vi "Safety_Check.vi"(1 "Adam Loop Count":i32, 2 "Ch Names":string[](array[string]), 3 "Values":dbl[](array[numeric]) format="%.2f") -> ()   [LabVIEW 2010]
uses:
  ADAM Client/Sub VIs/ADAM Controls/Update_scan_value.ctl
  Anemometry/Anemometry Sub Vis/Globals/Gas_management_global.vi
  ADAM_Global.vi
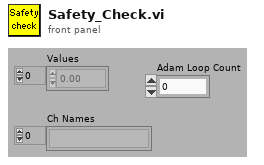
[diagram p1: front panel]
types:
  T1 = enum16{"On", "Off", "Always On", "Always Off", "Delete"}
  T2 = cluster{"Channel name":string, "Set value of A to":dbl, "Set value of B to":dbl, "Set value of C to":dbl, "Set value of D to":dbl}
  T3 = typedef "Update_scan_value.ctl" = cluster{"Channel Name":string, "New Value":dbl}
  T4 = enum16{"Append to Global", "Read Global then Clear"}
  T5 = typedef "LVDateTimeRec.ctl" = cluster{"fractional second":dbl, "second":i32, "minute":i32, "hour":i32, "day of month":i32, "month":i32, "year":i32, "day of week":i32, "day of year":i32, "DST":i32}
  T6 = cluster{"Channel name":string, "Set value of A to":dbl, "Set value of B to":dbl, "Set value of C to":dbl, "Set value of D to":dbl}[]
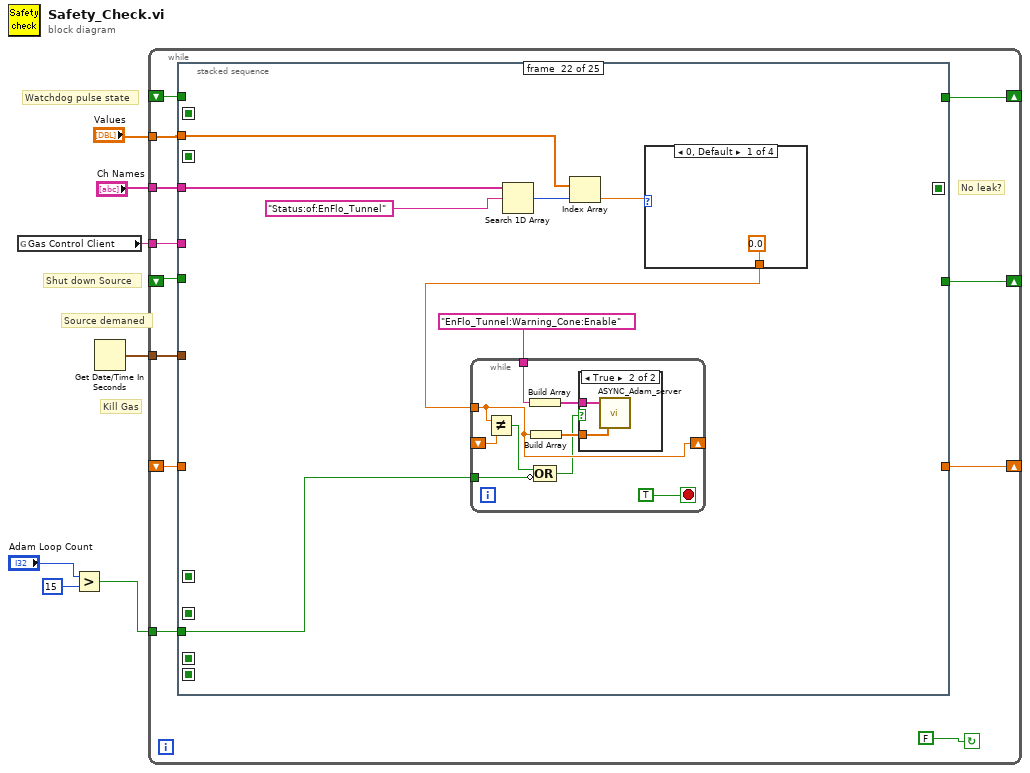
[diagram p0: block diagram]
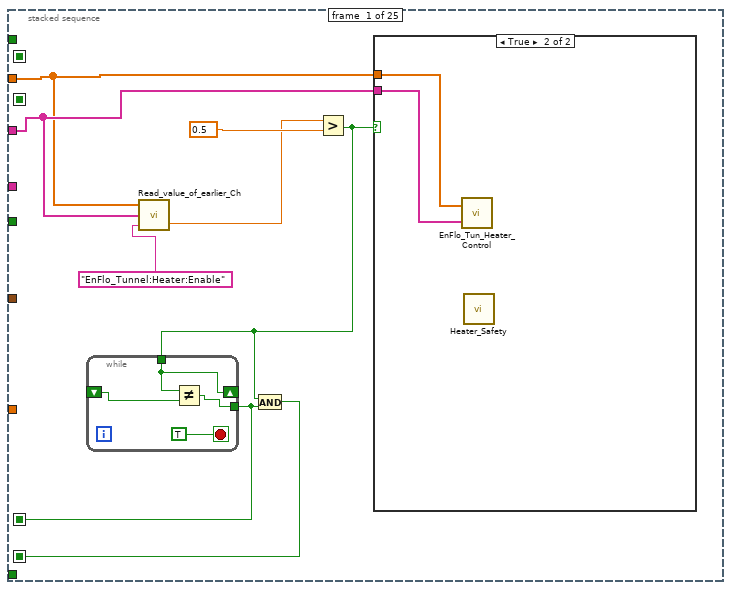
[diagram p2: hidden frame]
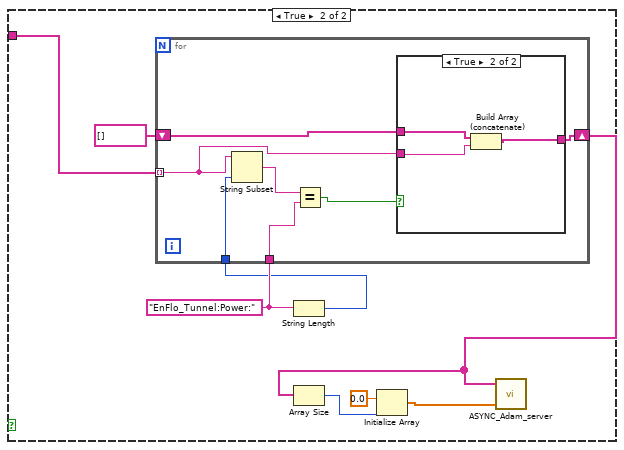
[diagram p5: hidden frame]
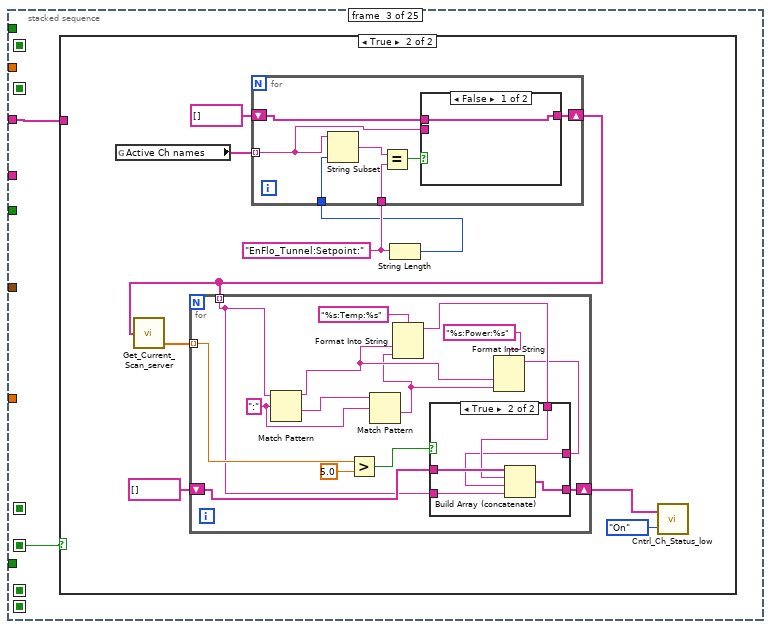
[diagram p7: hidden frame]
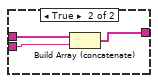
[diagram p10: hidden frame]
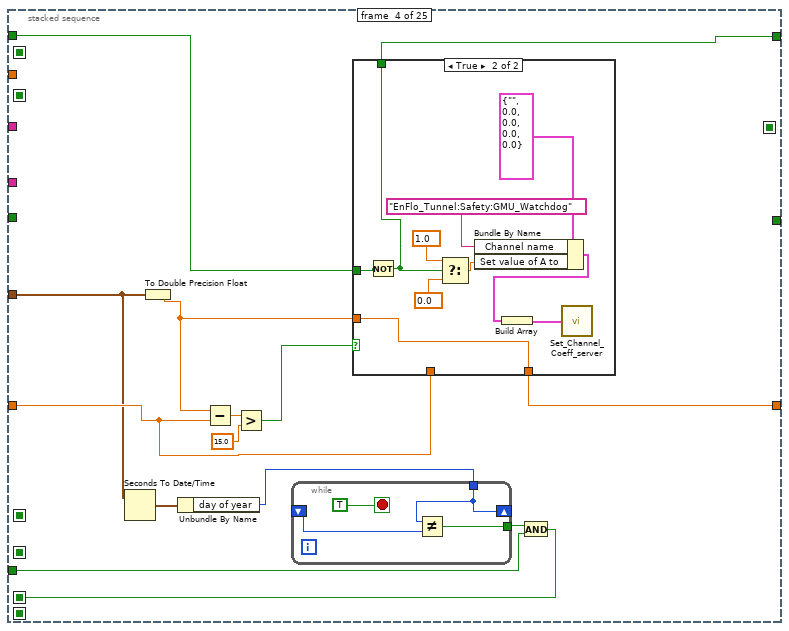
[diagram p11: hidden frame]
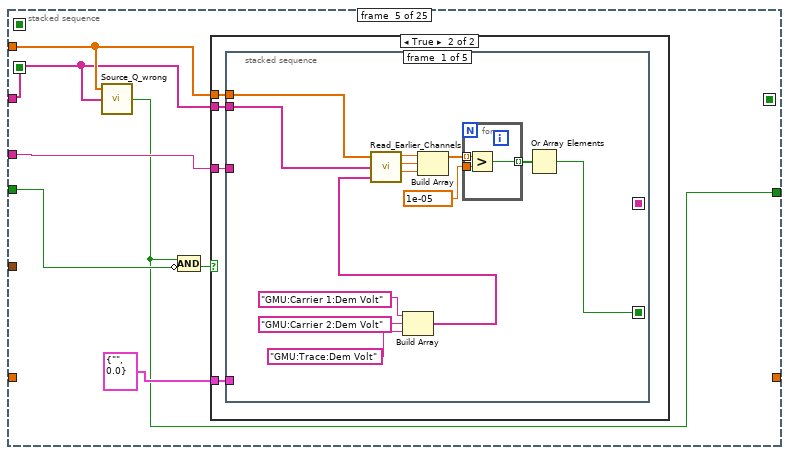
[diagram p13: hidden frame]
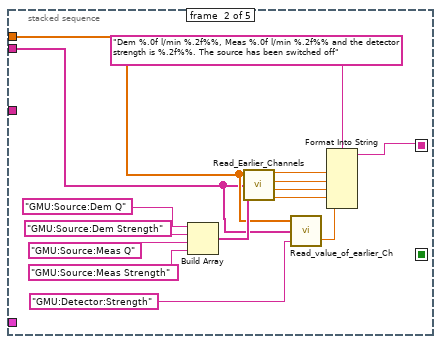
[diagram p15: hidden frame]
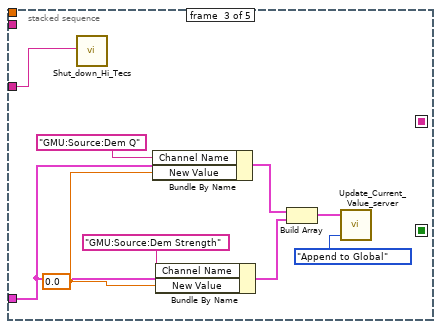
[diagram p16: hidden frame]
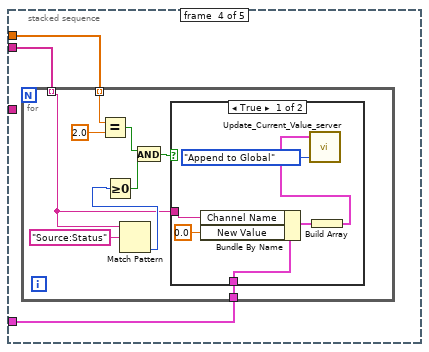
[diagram p17: hidden frame]
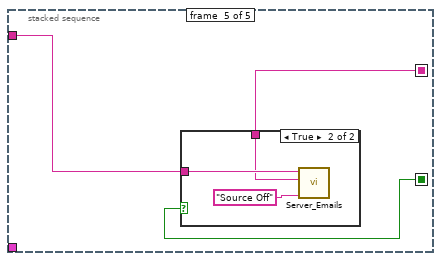
[diagram p19: hidden frame]
diagram:
  # "Shut down Source"
  # "Source demaned"
  # "Watchdog pulse state"
  # "Kill Gas"
  n1 = global read "Gas_management_global.vi" "Gas Control Client"() -> (w5:string)
  n2 = Greater?(x="Adam Loop Count", y=15) -> (0:w2:bool)
  n3 = Get Date/Time In Seconds() -> (seconds since 1Jan1904=w1:timestamp)
  n4 = while {
    shift-left: _ -> [w14]
    shift-right: [w13] -> _
    shift-left: _ -> [w16]
    shift-right: [w15] -> _
    tunnel: w5 -> [w18]
    tunnel: "Ch Names" -> [w19]
    tunnel: "Values" -> [w17]
    shift-right: [w11] -> _
    shift-left: _ -> [w10]
    tunnel: w2 -> [w9]
    tunnel: w1 -> [w8]
    stop <- FALSE continue-if-true
    # "No leak?"
    n5 = stacked-sequence {
      seq-local: [_ _ _ _ _ _ _ w234 _ _ _ _ _ _ _ _ _ _ _ _ _ _ _ _ _] -> [_ _ _ _ _ _ _ _ _ _ _ _ _ _ _ _ _ w505 _ _ _ _ _ _ _]
      seq-local: [w21 _ _ _ _ _ _ _ _ _ _ _ _ _ _ _ _ _ _ _ _ _ _ _ _] -> [_ _ w56 _ _ _ _ _ _ _ _ _ _ _ _ _ _ _ _ _ _ _ _ _ _]
      seq-local: [w20 _ _ _ _ _ _ _ _ _ _ _ _ _ _ _ _ _ _ _ _ _ _ _ _] -> [_ w34 _ _ _ _ _ _ _ _ _ _ _ _ _ _ _ _ _ _ _ _ _ _ _]
      seq-local: [_ _ _ w98 _ _ _ _ _ _ _ _ _ _ _ _ _ _ _ _ _ _ _ _ _] -> [_ _ _ _ _ _ _ _ _ _ _ _ _ _ _ w441 _ _ _ _ _ _ _ _ _]
      seq-local: [_ _ _ _ _ _ _ _ _ _ _ _ _ _ _ _ _ _ _ w534 _ _ _ _ _] -> [_ _ _ _ _ _ _ _ _ _ _ _ _ _ _ _ _ _ _ _ w560 _ _ _ _]
      seq-local: [_ _ _ _ _ _ _ _ _ _ _ _ _ _ _ _ _ _ _ _ w552 _ _ _ _] -> [_ _ _ _ _ _ _ _ _ _ _ _ _ _ _ _ _ _ _ _ _ _ _ w665 _]
      seq-local: [_ _ _ _ _ _ _ _ _ w276 _ _ _ _ _ _ _ _ _ _ _ _ _ _ _] -> [_ _ _ _ _ _ _ _ _ _ w303 _ _ _ _ _ _ _ _ _ _ _ _ _ _]
      tunnel: w19 -> [w25 w35 w55 _ w128 w207 w218 w235 w249 w277 _ w352 w380 w404 w423 w451 w476 w503 w521 w535 w561 w616 w635 _ w685]
      tunnel: w18 -> [_ _ _ _ w133 _ w217 _ _ _ _ _ _ _ _ _ _ _ _ _ _ _ _ _ _]
      tunnel: w17 -> [w24 _ _ _ w129 w203 w219 w236 w250 w278 _ w353 w381 w405 w424 w452 w477 w504 w522 w536 w562 w617 w636 _ w684]
      tunnel: w16 -> [_ _ _ w110 _ _ _ _ _ _ _ _ _ _ _ _ _ _ _ _ _ _ _ _ _]
      tunnel: [_ _ _ w109 _ _ _ _ _ _ _ _ _ _ _ _ _ _ _ _ _ _ _ _ _] -> w15
      tunnel: w14 -> [_ _ _ _ w132 _ _ _ _ _ _ _ _ _ _ _ _ _ _ _ _ _ _ _ _]
      tunnel: [_ _ _ _ w127 _ _ _ _ _ _ _ _ _ _ _ _ _ _ _ _ _ _ _ _] -> w13
      tunnel: [_ _ _ w108 _ _ _ _ _ _ _ _ _ _ _ _ _ _ _ _ _ _ _ _ _] -> w11
      tunnel: w10 -> [_ _ _ w104 _ _ _ _ _ _ _ _ _ _ _ _ _ _ _ _ _ _ _ _ _]
      tunnel: w9 -> [_ _ _ w99 _ _ _ _ _ _ w301 _ _ _ w422 _ _ _ _ _ w553 w612 _ w664 w679]
      tunnel: w8 -> [_ _ _ w97 _ _ _ _ _ _ w304 _ w376 _ _ _ _ _ _ _ _ _ _ _ _]
      frame #0 {
        n6 = call "Read_value_of_earlier_Ch.vi"("Desired Ch to Read"="EnFlo_Tunnel:Heater:Enable", "Ch names"=w25, "Present scan array"=w24) -> ("Value"=w23:dbl)  [unwired: 1 in, 1 out]
        n7 = Greater?(x=w23, y=0.5) -> (0:w22:bool)
        n8 = while {
          shift-right: [w31] -> _
          shift-left: _ -> [w30]
          tunnel: w22 -> [w31]
          tunnel: [w28] -> w20
          stop <- TRUE stop-if-true
          n9 = Not Equal?(x=w31, y=w30) -> (x != y?=w28:bool)
        }
        n10 = And(x=w22, y=w20) -> (x .and. y?=w21:bool)
        n11 = case shown="True" w22 {
          tunnel: w24 -> [_ w33]
          tunnel: w25 -> [_ w32]
          frame False {
          }
          frame True {
            n12 = call "EnFlo_Tun_Heater_Control.vi"("Ch Names"=w32, "Values"=w33) -> ()  [unwired: 1 out]
            n13 = call "Heater_Safety.vi"() -> ()  [unwired: 3 in, 5 out]
          }
        }
      }
      frame #1 {
        n14 = case shown="False" w34 {
          tunnel: w35 -> [_ w43]
          frame False {
          }
          frame True {
            w42 = "EnFlo_Tunnel:Power:"
            n15 = String Length(string=w42) -> (length=w41:i32)
            n16 = for {
              shift-right: [w45] -> w37
              shift-left: string[] [] -> [w46]
              tunnel: w43 -> [w49] mode=indexing
              tunnel: w41 -> [w50]
              tunnel: w42 -> [w47]
              n17 = String Subset(string=w49, length (rest)=w50) -> (substring=w48:string)  [unwired: 1 out]
              n18 = Equal?(x=w48, y=w47) -> (x = y?=w44:bool)
              n19 = case shown="True" w44 {
                tunnel: w49 -> [_ w54]
                tunnel: w46 -> [w51 w52]
                tunnel: [w51 w53] -> w45
                frame False {
                }
                frame True {
                  n20 = Build Array (concatenate)(w52, w54) -> (w53:string[])
                }
              }
            }
            n21 = Array Size(array=w37) -> (size(s)=w38:i32)
            n22 = Initialize Array(0.0 ("element"), w38) -> (w36:dbl[])
            n23 = call "ASYNC_Adam_server.vi"("Values"=w36, "Channel Names"=w37) -> ()  [unwired: 1 in, 3 out]
          }
        }
      }
      frame #2 {
        n24 = case shown="True" w56 {
          tunnel: w55 -> [_ _]
          frame False {
          }
          frame True {
            w64 = "EnFlo_Tunnel:Setpoint:"
            n25 = global read "ADAM_Global.vi" "Active Ch names"() -> (w62:string[])
            n26 = String Length(string=w64) -> (length=w63:i32)
            n27 = for {
              shift-right: [w86] -> w61
              shift-left: string[] [] -> [w88]
              tunnel: w62 -> [w87] mode=indexing
              tunnel: w63 -> [w92]
              tunnel: w64 -> [w91]
              n28 = String Subset(string=w87, length (rest)=w92) -> (substring=w90:string)  [unwired: 1 out]
              n29 = Equal?(x=w90, y=w91) -> (x = y?=w89:bool)
              n30 = case shown="False" w89 {
                tunnel: w88 -> [w93 w96]
                tunnel: w87 -> [_ w95]
                tunnel: [w93 w94] -> w86
                frame False {
                }
                frame True {
                  n31 = Build Array (concatenate)(w96, w95) -> (w94:string[])
                }
              }
            }
            n32 = call "Get_Current_Scan_server.vi"("Desired Channels"=w61) -> ("Numerical Values"=w60:dbl[])  [unwired: 2 out]
            n33 = for {
              tunnel: w61 -> [w66] mode=indexing
              tunnel: w60 -> [w73] mode=indexing
              shift-right: [w67] -> w58
              shift-left: string[] [] -> [w71]
              w78 = ":" ("regular expression")
              n34 = Match Pattern(string=w66, regular expression=w78) -> (before substring=w75:string, after substring=w79:string)  [unwired: 3 out]
              n35 = Greater?(x=w73, y=5.0) -> (0:w70:bool)
              n36 = Match Pattern(string=w79, regular expression=w78) -> (after substring=w74:string)  [unwired: 4 out]
              n37 = Format Into String(format string="%s:Temp:%s", w75, w74) -> (resulting string=w69:string)  [unwired: 2 in, 1 out]
              n38 = Format Into String(format string="%s:Power:%s", w75, w74) -> (resulting string=w68:string)  [unwired: 2 in, 1 out]
              n39 = case shown="True" w70 {
                tunnel: w71 -> [w80 w85]
                tunnel: w69 -> [_ w84]
                tunnel: w68 -> [_ w83]
                tunnel: [w80 w82] -> w67
                tunnel: w66 -> [_ w81]
                frame False {
                }
                frame True {
                  n40 = Build Array (concatenate)(w85, w84, w83, w81) -> (w82:string[])
                }
              }
            }
            n41 = call "Cntrl_Ch_Status_low.vi"("Mode"=T1."On", "Channel names"=w58) -> ()  [unwired: 1 out]
          }
        }
      }
      frame #3 {
        n42 = Seconds To Date/Time(time stamp (now)=w97) -> (date time rec=w102:T5)  [unwired: 1 in]
        n43 = To Double Precision Float(number=w97) -> (double precision float=w107:dbl)
        n44 = Unbundle By Name(w102) -> ("day of year"=w101:i32)
        n45 = Subtract(x=w107, y=w104) -> (x-y=w106:dbl)
        n46 = Greater?(x=w106, y=15.0) -> (0:w103:bool)
        n47 = while {
          shift-right: [w114] -> _
          shift-left: _ -> [w113]
          tunnel: w101 -> [w114]
          tunnel: [w112] -> w100
          stop <- TRUE stop-if-true
          n48 = Not Equal?(x=w114, y=w113) -> (x != y?=w112:bool)
        }
        n49 = case shown="True" w103 {
          tunnel: w110 -> [w115 w119]
          tunnel: [w115 w118] -> w109
          tunnel: [w116 w117] -> w108
          tunnel: w107 -> [_ w117]
          tunnel: w104 -> [w116 _]
          frame False {
          }
          frame True {
            n50 = Not(x=w119) -> (.not. x?=w118:bool)
            n51 = Select(t=1.0 ("Suction"), s=w118, f=0.0 ("Suction")) -> (s? t:f=w122:dbl)
            n52 = Bundle By Name(cluster=T2 {"Channel name"="", "Set value of A to"=0.0, "Set value of B to"=0.0, "Set value of C to"=0.0, "Set value of D to"=0.0}, "Channel name"="EnFlo_Tunnel:Safety:GMU_Watchdog" ("Desired Ch to Read"), "Set value of A to"=w122) -> (w126:T2)
            n53 = Build Array(w126) -> (w121:T6)
            n54 = call "Set_Channel_Coeff_server.vi"("Set Array"=w121) -> ()
          }
        }
        n55 = And(x=w100, y=w99) -> (x .and. y?=w98:bool)
      }
      frame #4 {
        n56 = call "Source_Q_wrong.vi"("Ch Names"=w128, "Values"=w129) -> ("Gas Error?"=w127:bool)  [unwired: 1 out]
        n57 = Compound Arithmetic op=AND(w127, invert w132) -> (w131:bool)
        n58 = case shown="True" w131 {
          tunnel: w133 -> [_ w137]
          tunnel: w129 -> [_ w136]
          tunnel: w128 -> [_ w135]
          tunnel: T3 {"Channel Name"="", "New Value"=0.0} ("Update Scan Value Cluster") -> [_ w134]
          frame False {
          }
          frame True {
            n59 = stacked-sequence {
              seq-local: [_ w167 _ _ _] -> [_ _ _ _ w197]
              seq-local: [w138 _ _ _ _] -> [_ _ _ _ w196]
              tunnel: w137 -> [_ _ w170 _ w198]
              tunnel: w136 -> [w148 w157 _ w179 _]
              tunnel: w135 -> [w149 w156 _ w180 _]
              tunnel: w134 -> [_ _ w169 w178 _]
              frame #0 {
                n60 = Build Array("GMU:Carrier 1:Dem Volt", "GMU:Carrier 2:Dem Volt", "GMU:Trace:Dem Volt") -> (w150:string[])
                n61 = call "Read_Earlier_Channels.vi"("Present scan array"=w148, "Ch names"=w149, "Desired Channels"=w150) -> ("Index 0"=w144:dbl, "Index 1"=w143:dbl, "Index 2"=w142:dbl)  [unwired: 3 out]
                n62 = Build Array(w144, w143, w142) -> (w141:dbl[])
                n63 = for {
                  tunnel: w141 -> [w153] mode=indexing
                  tunnel: 1e-05 -> [w152]
                  tunnel: [w151] -> w139 mode=indexing
                  n64 = Greater?(x=w153, y=w152) -> (0:w151:bool)
                }
                n65 = Or Array Elements(Boolean array=w139) -> (logical OR=w138:bool)
              }
              frame #1 {
                n66 = Build Array("GMU:Source:Dem Q", "GMU:Source:Dem Strength", "GMU:Source:Meas Q", "GMU:Source:Meas Strength") -> (w162:string[])
                n67 = call "Read_Earlier_Channels.vi"("Present scan array"=w157, "Ch names"=w156, "Desired Channels"=w162) -> ("Index 0"=w161:dbl, "Index 1"=w160:dbl, "Index 2"=w159:dbl, "Index 3"=w158:dbl)  [unwired: 2 out]
                n68 = call "Read_value_of_earlier_Ch.vi"("Desired Ch to Read"="GMU:Detector:Strength", "Ch names"=w156, "Present scan array"=w157) -> ("Value"=w154:dbl)  [unwired: 1 in, 1 out]
                n69 = Format Into String(format string="Dem %.0f l/min %.2f%%, Meas %.0f l/min %.2f%% and the detector strength is %.2f%%. The source has been switched off" ("Format String"), w161, w160, w159, w158, w154) -> (resulting string=w167:string)  [unwired: 2 in, 1 out]
              }
              frame #2 {
                w171 = 0.0 ("Bundle Element")
                n70 = call "Shut_down_Hi_Tecs.vi"("Client Name"=w170) -> ()  [unwired: 6 out]
                n71 = Bundle By Name(cluster=w169, "Channel Name"="GMU:Source:Dem Q", "New Value"=w171) -> (w176:T3)
                n72 = Bundle By Name(cluster=w169, "Channel Name"="GMU:Source:Dem Strength", "New Value"=w171) -> (w177:T3)
                n73 = Build Array(w176, w177) -> (w173:T3[])
                n74 = call "Update_Current_Value_server.vi"("Mode"=T4."Append to Global", "Update array in"=w173) -> ()  [unwired: 1 in, 1 out]
              }
              frame #3 {
                n75 = for {
                  tunnel: w180 -> [w181] mode=indexing
                  tunnel: w179 -> [w187] mode=indexing
                  tunnel: w178 -> [w182]
                  n76 = Equal?(x=w187, y=2.0) -> (x = y?=w184:bool)
                  n77 = Match Pattern(string=w181, regular expression="Source:Status") -> (offset past match=w188:i32)  [unwired: 4 out]
                  n78 = Greater Or Equal To 0?(x=w188) -> (x >= 0?=w185:bool)
                  n79 = And(x=w184, y=w185) -> (x .and. y?=w183:bool)
                  n80 = case shown="True" w183 {
                    tunnel: w182 -> [w195 _]
                    tunnel: w181 -> [w194 _]
                    frame True {
                      n81 = Bundle By Name(cluster=w195, "Channel Name"=w194, "New Value"=0.0) -> (w192:T3)
                      n82 = Build Array(w192) -> (w191:T3[])
                      n83 = call "Update_Current_Value_server.vi"("Mode"=T4."Append to Global", "Update array in"=w191) -> ()  [unwired: 1 in, 1 out]
                    }
                    frame False {
                    }
                  }
                }
              }
              frame #4 {
                n84 = case shown="True" w196 {
                  tunnel: w198 -> [_ w201]
                  tunnel: w197 -> [_ w200]
                  frame False {
                  }
                  frame True {
                    n85 = call "Server_Emails.vi"("Client Name Contains"=w201, "Message"=w200, "Subject"="Source Off") -> ()  [unwired: 2 in, 3 out]
                  }
                }
              }
            }
          }
        }
      }
      frame #5 {
        n86 = global read "ADAM_Global.vi" "Program Hung Clients"() -> (w208:string[])
        n87 = for {
          tunnel: w208 -> [w214] mode=indexing
          tunnel: w203 -> [w216]
          tunnel: w207 -> [w215]
          tunnel: [w212] -> w206 mode=indexing
          tunnel: [w209] -> w205 mode=indexing
          n88 = call "Split_Ch_name.vi"("Ch name"=w214) -> ("Low level"=w211:string)  [unwired: 2 out]
          n89 = call "Shut_Down_Client_Demands.vi"("Ch Names"=w215, "Values"=w216, "Client Name"=w214) -> ()  [unwired: 1 out]
          n90 = Concatenate Strings(w211, ":Source:Status") -> (w212:string)
          n91 = Concatenate Strings(w211, ":Program:Sync") -> (w209:string)
        }
        n92 = Build Array (concatenate)(w206, w205) -> (w204:string[])
        n93 = call "Cntrl_Ch_Status_low.vi"("Mode"=T1."Delete", "Channel names"=w204) -> ()  [unwired: 1 out]
      }
      frame #6 {
        n94 = while {
          tunnel: w219 -> [w230]
          tunnel: w218 -> [w229]
          shift-right: [w224] -> _
          shift-left: _ -> [w225]
          tunnel: w217 -> [w222]
          stop <- FALSE continue-if-true
          n95 = call "Read_value_of_earlier_Ch.vi"("Desired Ch to Read"="GMU:Detector:Happy", "Ch names"=w229, "Present scan array"=w230) -> ("Value"=w227:dbl)  [unwired: 1 in, 1 out]
          n96 = Greater?(x=w227, y=0.5) -> (0:w224:bool)
          n97 = Compound Arithmetic op=AND(invert w224, w225) -> (w223:bool)
          n98 = case shown="True" w223 {
            tunnel: w222 -> [_ w232]
            frame False {
            }
            frame True {
              n99 = call "Server_Emails.vi"("Client Name Contains"=w232, "Message"="The GMU Gas detector IR2100 is unhappy. Please check concentrations etc. This will have turned off the gases from the outside bottle store.  You will need to repress the blue gas button after clearing the fault by purging the source with carrier gas only.", "Subject"="GMU Gas Detector Unhappy") -> ()  [unwired: 2 in, 3 out]
            }
          }
        }
        n100 = global write "ADAM_Global.vi" "Program Hung Clients"(string[] [] ("Program Hung Clients")) -> ()
      }
      frame #7 {
        n101 = while {
          tunnel: w236 -> [w245]
          tunnel: w235 -> [w244]
          shift-right: [w239] -> w234
          shift-left: _ -> [w240]
          stop <- FALSE continue-if-true
          n102 = call "Read_value_of_earlier_Ch.vi"("Desired Ch to Read"="EnFlo Lab:Leak_Detector:Happy", "Ch names"=w244, "Present scan array"=w245) -> ("Value"=w242:dbl)  [unwired: 1 in, 1 out]
          n103 = Greater?(x=w242, y=0.5) -> (0:w239:bool)
          n104 = Compound Arithmetic op=AND(invert w239, w240) -> (w238:bool)
          n105 = case shown="True" w238 {
            frame False {
            }
            frame True {
              n106 = call "Server_Emails.vi"("Client Name Contains"="EnFlo_Tunnel", "Message"="The leak detector is indicating a leak under the Enflo Tunnel. The chiller pumps should automaticaly be turned off and the cooling circuit isolated from the  University Chilled water system. The heaters should also have been disabled.", "Subject"="Leak Detected under EnFlo Tunnel") -> ()  [unwired: 2 in, 3 out]
            }
          }
        }
      }
      frame #8 {
        n107 = while {
          tunnel: w250 -> [w262]
          tunnel: w249 -> [w261]
          shift-right: [w255] -> _
          shift-left: _ -> [w251]
          stop <- FALSE continue-if-true
          w253 = 60.0 ("y")
          n108 = Decrement(x=w253) -> (x-1=w254:dbl)
          n109 = Select(t=w254, s=w251, f=w253) -> (s? t:f=w252:dbl)
          n110 = call "Read_value_of_earlier_Ch.vi"("Desired Ch to Read"="EnFlo_Tunnel:Chilled Water:Motor1 Temp", "Ch names"=w261, "Present scan array"=w262) -> ("Value"=w269:dbl)  [unwired: 1 in, 1 out]
          n111 = call "Read_value_of_earlier_Ch.vi"("Desired Ch to Read"="EnFlo_Tunnel:Chilled Water:Motor2 Temp", "Ch names"=w261, "Present scan array"=w262) -> ("Value"=w266:dbl)  [unwired: 1 in, 1 out]
          n112 = Greater?(x=w269, y=w252) -> (0:w263:bool)
          n113 = Greater?(x=w266, y=w252) -> (0:w264:bool)
          n114 = Or(x=w263, y=w264) -> (x .or. y?=w257:bool)
          n115 = call "Read_value_of_earlier_Ch.vi"("Desired Ch to Read"="EnFlo_Tunnel:Chiller_Pump:Enable", "Ch names"=w261, "Present scan array"=w262) -> ("Value"=w259:dbl)  [unwired: 1 in, 1 out]
          n116 = Greater?(x=w259, y=0.5) -> (0:w256:bool)
          n117 = And(x=w256, y=w257) -> (x .and. y?=w255:bool)
          n118 = Compound Arithmetic op=AND(w255, invert w251) -> (w268:bool)
          n119 = case shown="True" w268 {
            tunnel: w253 -> [_ w272]
            frame False {
            }
            frame True {
              n120 = Format Into String(format string="The Chilled Water Motor Temp is greater than %.0f deg C." ("Message"), w272) -> (resulting string=w271:string)  [unwired: 2 in, 1 out]
              n121 = call "Server_Emails.vi"("Client Name Contains"="EnFlo_Tunnel", "Message"=w271, "Subject"="Chilled Water Motor Temp") -> ()  [unwired: 2 in, 3 out]
            }
          }
        }
      }
      frame #9 {
        n122 = while {
          tunnel: w278 -> [w291]
          tunnel: w277 -> [w290]
          shift-right: [w286] -> _
          shift-left: _ -> [w283]
          tunnel: [w279] -> w276
          stop <- FALSE continue-if-true
          w281 = 60.0 ("y")
          w284 = "Laser:Cooling_Pump:Motor_Temp" ("Desired Ch to Read")
          n123 = Decrement(x=w281) -> (x-1=w280:dbl)
          n124 = Select(t=w280, s=w283, f=w281) -> (s? t:f=w282:dbl)
          n125 = call "Read_value_of_earlier_Ch.vi"("Desired Ch to Read"=w284, "Ch names"=w290, "Present scan array"=w291) -> ("Value"=w294:dbl)  [unwired: 1 in, 1 out]
          n126 = Greater?(x=w294, y=w282) -> (0:w285:bool)
          n127 = call "Read_value_of_earlier_Ch.vi"("Desired Ch to Read"="Laser:Cooling_Pump:Enable", "Ch names"=w290, "Present scan array"=w291) -> ("Value"=w288:dbl)  [unwired: 1 in, 1 out]
          n128 = Greater?(x=w288, y=0.5) -> (0:w279:bool)
          n129 = And(x=w279, y=w285) -> (x .and. y?=w286:bool)
          n130 = Compound Arithmetic op=AND(w286, invert w283) -> (w293:bool)
          n131 = case shown="True" w293 {
            tunnel: w281 -> [_ w297]
            tunnel: w284 -> [_ w295]
            frame False {
            }
            frame True {
              n132 = Format Into String(format string="The %s is greater than %.0f deg C." ("Message"), w295, w297) -> (resulting string=w296:string)  [unwired: 2 in, 1 out]
              n133 = call "Server_Emails.vi"("Client Name Contains"="EnFlo_Tunnel", "Message"=w296, "Subject"=w295) -> ()  [unwired: 2 in, 3 out]
            }
          }
        }
      }
      frame #10 {
        n134 = case shown="True" w303 {
          tunnel: w304 -> [_ w338]
          tunnel: [0.0 ("y") w323] -> w300
          frame False {
          }
          frame True {
            w336 = 7200.0  # Seconds
            w334 = FALSE  # All Active Channels
            n135 = To Double Precision Float(number=w338) -> (double precision float=w332:dbl)
            n136 = call "Channel_Names_and_indicies.vi"("All Active Channels"=w334, "Desired Ch Names"=string[] ["LDA Laser:Tank:Supply Temp", "LDA Laser:Tank:Return Temp"]) -> ("Indicies"=w335:i32[])  [unwired: 1 out]
            n137 = Subtract(x=w332, y=w336) -> (x-y=w337:dbl)
            n138 = call "Specified_Channels_server.vi"("End time"=w332, "Start time"=w337, "Clients time"=w332, "Requested channels"=w335) -> ("Output array"=w329:dbl[][])  [unwired: 1 in, 4 out]
            n139 = Index Array(array=w329, index (row)=1) -> (element=w328:dbl[])  [unwired: 1 in]
            n140 = Index Array(array=w329, index (row)=0) -> (element=w327:dbl[])  [unwired: 1 in]
            n141 = Subtract(x=w328, y=w327) -> (x-y=w318:dbl[])
            n142 = Not A Number/Path/Refnum?(number/path/refnum=w318) -> (NaN/Path/Refnum?=w319:bool[])
            n143 = Or Array Elements(Boolean array=w319) -> (logical OR=w320:bool)
            n144 = case shown="True" w320 {
              tunnel: w319 -> [_ w343]
              tunnel: w318 -> [w339 w342]
              tunnel: [w339 w340] -> w317
              frame False {
              }
              frame True {
                n145 = for {
                  shift-right: [w346] -> w340
                  shift-left: dbl[] [] -> [w345]
                  tunnel: w343 -> [w347] mode=indexing
                  tunnel: w342 -> [w344] mode=indexing
                  n146 = case shown="True" w347 {
                    tunnel: [w349 w351] -> w346
                    tunnel: w345 -> [w350 w351]
                    tunnel: w344 -> [w348 _]
                    frame False {
                      n147 = Build Array (concatenate)(w350, w348) -> (w349:dbl[])
                    }
                    frame True {
                    }
                  }
                }
              }
            }
            n148 = Greater?(x=w317, y=3.0) -> (0:w322:bool[])
            n149 = And Array Elements(Boolean array=w322) -> (logical AND=w321:bool)
            n150 = Select(t=1.0 ("y"), s=w321, f=0.0 ("y")) -> (s? t:f=w323:dbl)
          }
        }
        n151 = while {
          shift-right: [w309] -> _
          shift-left: _ -> [w310]
          tunnel: w300 -> [w309]
          tunnel: "LDA:Full_Power:Enable" -> [w311]
          tunnel: w301 -> [w306]
          stop <- TRUE stop-if-true
          n152 = Not Equal?(x=w309, y=w310) -> (x != y?=w307:bool)
          n153 = Compound Arithmetic op=OR(w307, invert w306) -> (w305:bool)
          n154 = Build Array(w311) -> (w312:string[])
          n155 = Build Array(w309) -> (w313:dbl[])
          n156 = case shown="True" w305 {
            tunnel: w313 -> [_ w315]
            tunnel: w312 -> [_ w314]
            frame False {
            }
            frame True {
              n157 = call "ASYNC_Adam_server.vi"("Values"=w315, "Channel Names"=w314) -> ()  [unwired: 1 in, 3 out]
            }
          }
        }
      }
      frame #11 {
        n158 = while {
          tunnel: w353 -> [w366]
          tunnel: w352 -> [w365]
          shift-right: [w354] -> _
          shift-left: _ -> [w360]
          shift-left: _ -> [w359]
          shift-left: _ -> [w358]
          stop <- FALSE continue-if-true
          n159 = call "Read_value_of_earlier_Ch.vi"("Desired Ch to Read"="LDA:System:Enable", "Ch names"=w365, "Present scan array"=w366) -> ("Value"=w361:dbl)  [unwired: 1 in, 1 out]
          n160 = Greater?(x=w361, y=0.5) -> (0:w354:bool)
          n161 = Compound Arithmetic op=AND(w354, w360, invert w359, invert w358) -> (w356:bool)
          n162 = Compound Arithmetic op=AND(invert w354, invert w360, w359, w358) -> (w357:bool)
          n163 = Or(x=w356, y=w357) -> (x .or. y?=w355:bool)
          n164 = case shown="True" w355 {
            tunnel: w361 -> [_ w367]
            tunnel: w354 -> [_ w371]
            frame False {
            }
            frame True {
              n165 = case shown="True" w371 {
                tunnel: [string[] ["LDA:3 Phase:Power", "Hydrosonic:Seeder:Enable", "Laser:Cooling_Pump:Enable"] ("Channel Names") string[] ["LDA:3 Phase:Power", "Hydrosonic:Seeder:Enable"] ("Channel Names")] -> w370
                frame True {
                }
                frame False {
                }
              }
              n166 = Array Size(array=w370) -> (size(s)=w368:i32)
              n167 = Initialize Array(w367, w368) -> (w369:dbl[])
              n168 = call "ASYNC_Adam_server.vi"("Values"=w369, "Channel Names"=w370) -> ()  [unwired: 1 in, 3 out]
            }
          }
        }
      }
      frame #12 {
        w375 = "Hydrosonic:Seeder:Enable" ("Desired Ch to Read")
        # "This turns the Hydrosonic off for 20 seconds each hour which appears to help it."
        n169 = call "Read_value_of_earlier_Ch.vi"("Desired Ch to Read"=w375, "Ch names"=w380, "Present scan array"=w381) -> ("Value"=w378:dbl)  [unwired: 1 in, 1 out]
        n170 = Greater?(x=w378, y=0.2) -> (0:w377:bool)
        n171 = case shown="True" w377 {
          tunnel: w378 -> [w391 _]
          tunnel: w376 -> [_ w402]
          tunnel: [w391 w392] -> w374
          frame False {
          }
          frame True {
            n172 = Seconds To Date/Time(time stamp (now)=w402) -> (date time rec=w403:T5)  [unwired: 1 in]
            n173 = Unbundle By Name(w403) -> ("minute"=w401:i32, "second"=w399:i32)
            n174 = Equal?(x=1, y=w401) -> (x = y?=w396:bool)
            n175 = Less?(x=w399, y=20) -> (x < y?=w397:bool)
            n176 = And(x=w396, y=w397) -> (x .and. y?=w395:bool)
            n177 = Select(t=0.3 ("y"), s=w395, f=1.0) -> (s? t:f=w392:dbl)
          }
        }
        n178 = while {
          shift-right: [w384] -> _
          shift-left: _ -> [w385]
          tunnel: w374 -> [w384]
          tunnel: w375 -> [w386]
          stop <- TRUE stop-if-true
          n179 = Not Equal?(x=w384, y=w385) -> (x != y?=w382:bool)
          n180 = Build Array(w386) -> (w387:string[])
          n181 = Build Array(w384) -> (w388:dbl[])
          n182 = case shown="True" w382 {
            tunnel: w388 -> [_ w390]
            tunnel: w387 -> [_ w389]
            frame False {
            }
            frame True {
              n183 = call "ASYNC_Adam_server.vi"("Values"=w390, "Channel Names"=w389) -> ()  [unwired: 1 in, 3 out]
            }
          }
        }
      }
      frame #13 {
        n184 = while {
          tunnel: w405 -> [w418]
          tunnel: w404 -> [w417]
          shift-right: [w406] -> _
          shift-left: _ -> [w412]
          shift-left: _ -> [w411]
          shift-left: _ -> [w410]
          stop <- FALSE continue-if-true
          n185 = call "Read_value_of_earlier_Ch.vi"("Desired Ch to Read"="FFID:System:Enable", "Ch names"=w417, "Present scan array"=w418) -> ("Value"=w413:dbl)  [unwired: 1 in, 1 out]
          n186 = Greater?(x=w413, y=0.5) -> (0:w406:bool)
          n187 = Compound Arithmetic op=AND(w406, w412, invert w411, invert w410) -> (w408:bool)
          n188 = Compound Arithmetic op=AND(invert w406, invert w412, w411, w410) -> (w409:bool)
          n189 = Or(x=w408, y=w409) -> (x .or. y?=w407:bool)
          n190 = case shown="True" w407 {
            tunnel: w413 -> [_ w419]
            tunnel: w406 -> [_ _]
            frame False {
            }
            frame True {
              n191 = Build Array(w419) -> (w421:dbl[])
              n192 = call "ASYNC_Adam_server.vi"("Values"=w421, "Channel Names"=string[] ["GMU:Gas:Enable"]) -> ()  [unwired: 1 in, 3 out]
            }
          }
        }
      }
      frame #14 {
        # "Resetting A Tunnel speed to zero if the drive in turned off\nso that the belts do not slip when the tunnel is turned on again."
        n193 = while {
          tunnel: w424 -> [w436]
          tunnel: w423 -> [w435]
          shift-right: [w427] -> _
          shift-left: _ -> [w430]
          shift-left: _ -> [w429]
          shift-left: _ -> [w428]
          tunnel: w422 -> [w426]
          stop <- FALSE continue-if-true
          n194 = call "Read_value_of_earlier_Ch.vi"("Desired Ch to Read"="A_Tunnel:Motor:Enable", "Ch names"=w435, "Present scan array"=w436) -> ("Value"=w431:dbl)  [unwired: 1 in, 1 out]
          n195 = Less?(x=w431, y=0.5) -> (x < y?=w427:bool)
          n196 = Compound Arithmetic op=AND(w427, w430, invert w429, invert w428, w426) -> (w425:bool)
          n197 = case shown="True" w425 {
            tunnel: w427 -> [_ _]
            frame False {
            }
            frame True {
              w439 = string[] ["A_Tunnel:Speed:Dem Velocity", "A_Tunnel:Speed:Dem Voltage"] ("Channel Names")
              n198 = Array Size(array=w439) -> (size(s)=w440:i32)
              n199 = Initialize Array(0.0 ("element"), w440) -> (w438:dbl[])
              n200 = call "ASYNC_Adam_server.vi"("Values"=w438, "Channel Names"=w439) -> ()  [unwired: 1 in, 3 out]
            }
          }
        }
      }
      frame #15 {
        w445 = "LDA:3 Phase:Power" ("Desired Ch to Read")
        w450 = 0.5 ("y")
        w444 = "Laser:Cooling_Pump:Enable" ("Desired Ch to Read")
        n201 = call "Read_value_of_earlier_Ch.vi"("Desired Ch to Read"=w445, "Ch names"=w451, "Present scan array"=w452) -> ("Value"=w449:dbl)  [unwired: 1 in, 1 out]
        n202 = call "Read_value_of_earlier_Ch.vi"("Desired Ch to Read"=w444, "Ch names"=w451, "Present scan array"=w452) -> ("Value"=w453:dbl)  [unwired: 1 in, 1 out]
        n203 = Less?(x=w449, y=w450) -> (x < y?=w448:bool)
        n204 = Greater?(x=w453, y=w450) -> (0:w447:bool)
        n205 = And(x=w448, y=w447) -> (x .and. y?=w446:bool)
        n206 = case shown="True" w446 {
          tunnel: w445 -> [_ w462]
          tunnel: w444 -> [_ _]
          tunnel: [w458 w461] -> w443
          tunnel: [1.0 ("element") 0.0 ("element")] -> w442
          tunnel: w441 -> [w458 _]
          frame False {
          }
          frame True {
            n207 = Build Array(w462) -> (w467:string[])
            n208 = call "Get_Channel_averages.vi"("Desired Ch Names"=w467, "Averaging time (mins)"=20.0) -> ("number"=w466:dbl[])  [unwired: 1 in, 2 out]
            n209 = Index Array(array=w466, index=0) -> (element=w464:dbl)
            n210 = Less?(x=w464, y=0.02) -> (x < y?=w461:bool)
          }
        }
        n211 = case shown="False" w443 {
          tunnel: w444 -> [_ w455]
          tunnel: w442 -> [_ w454]
          frame False {
          }
          frame True {
            n212 = Build Array(w455) -> (w456:string[])
            n213 = Build Array(w454) -> (w457:dbl[])
            n214 = call "ASYNC_Adam_server.vi"("Values"=w457, "Channel Names"=w456) -> ()  [unwired: 1 in, 3 out]
          }
        }
      }
      frame #16 {
        w469 = "Laser:Cooling_Pump:Motor_Temp" ("Desired Ch to Read")
        w472 = "Laser:Cooling_Pump:Enable" ("Desired Ch to Read")
        n215 = call "Read_value_of_earlier_Ch.vi"("Desired Ch to Read"=w469, "Ch names"=w476, "Present scan array"=w477) -> ("Value"=w471:dbl)  [unwired: 1 in, 1 out]
        n216 = call "Read_value_of_earlier_Ch.vi"("Desired Ch to Read"=w472, "Ch names"=w476, "Present scan array"=w477) -> ("Value"=w478:dbl)  [unwired: 1 in, 1 out]
        n217 = Greater?(x=w478, y=0.5) -> (0:w474:bool)
        n218 = while {
          shift-right: [w483] -> _
          shift-left: _ -> [_]
          shift-left: _ -> [_]
          shift-left: _ -> [_]
          shift-left: _ -> [_]
          shift-left: _ -> [w482]
          tunnel: w471 -> [w483]
          tunnel: [w479] -> w470
          stop <- TRUE stop-if-true
          n219 = Subtract(x=w483, y=w482) -> (x-y=w481:dbl)
          n220 = Greater?(x=w481, y=2.0) -> (0:w479:bool)
        }
        n221 = And(x=w470, y=w474) -> (x .and. y?=w473:bool)
        n222 = case shown="True" w473 {
          tunnel: w472 -> [_ w486]
          tunnel: w469 -> [_ w485]
          frame False {
          }
          frame True {
            n223 = Build Array(w486) -> (w492:string[])
            n224 = call "Get_Channel_averages.vi"("Desired Ch Names"=w492, "Averaging time (mins)"=1.0) -> ("number"=w491:dbl[])  [unwired: 1 in, 2 out]
            n225 = Index Array(array=w491, index=0) -> (element=w489:dbl)
            n226 = Less?(x=w489, y=0.4) -> (x < y?=w487:bool)
            n227 = case shown="True" w487 {
              tunnel: w486 -> [_ w495]
              tunnel: w485 -> [_ w496]
              frame False {
              }
              frame True {
                n228 = Format Into String(format string="The %s is rising rapidly and may indicate that the motor is  seized. %s has therefore been set to zero. You should be able to unseized the motor by turning the motor shaft with a screw driver to loosen it up.", w496, w495) -> (resulting string=w494:string)  [unwired: 2 in, 1 out]
                n229 = Build Array(w495) -> (w500:string[])
                n230 = Build Array(0.0 ("element")) -> (w502:dbl[])
                n231 = call "ASYNC_Adam_server.vi"("Values"=w502, "Channel Names"=w500) -> ()  [unwired: 1 in, 3 out]
                n232 = call "Server_Emails.vi"("Client Name Contains"="EnFlo_Tunnel", "Message"=w494, "Subject"="Laser cooling Pump") -> ()  [unwired: 2 in, 3 out]
              }
            }
          }
        }
      }
      frame #17 {
        n233 = case shown="False" w505 {
          tunnel: w504 -> [w508 _]
          tunnel: w503 -> [w507 _]
          frame False {
            n234 = for {
              tunnel: w508 -> [w514]
              tunnel: w507 -> [w513]
              tunnel: string[] ["EnFlo_Tunnel:Heater:Enable", "EnFlo_Tunnel:Chiller_Pump:Enable", "EnFlo_Tunnel:Tap_Water:Enable"] ("Ch Names") -> [w509] mode=indexing
              n235 = call "Read_value_of_earlier_Ch.vi"("Desired Ch to Read"=w509, "Ch names"=w513, "Present scan array"=w514) -> ("Value"=w511:dbl)  [unwired: 1 in, 1 out]
              n236 = Greater?(x=w511, y=0.5) -> (0:w510:bool)
              n237 = case shown="True" w510 {
                tunnel: w509 -> [_ w515]
                frame False {
                }
                frame True {
                  n238 = Build Array(w515) -> (w518:string[])
                  n239 = Build Array(0.0) -> (w517:dbl[])
                  n240 = call "ASYNC_Adam_server.vi"("Values"=w517, "Channel Names"=w518) -> ()  [unwired: 1 in, 3 out]
                }
              }
            }
          }
          frame True {
          }
        }
      }
      frame #18 {
        w523 = "EnFlo_Tunnel:Heater:Enable" ("Ch Name")
        n241 = call "Read_value_of_earlier_Ch.vi"("Desired Ch to Read"=w523, "Ch names"=w521, "Present scan array"=w522) -> ("Value"=w528:dbl)  [unwired: 1 in, 1 out]
        n242 = call "Read_value_of_earlier_Ch.vi"("Desired Ch to Read"="EnFlo_Tunnel:Reference:Velocity", "Ch names"=w521, "Present scan array"=w522) -> ("Value"=w525:dbl)  [unwired: 1 in, 1 out]
        n243 = Greater?(x=w528, y=0.5) -> (0:w520:bool)
        n244 = Less?(x=w525, y=0.25) -> (x < y?=w524:bool)
        n245 = And(x=w520, y=w524) -> (x .and. y?=w519:bool)
        n246 = case shown="True" w519 {
          tunnel: w523 -> [_ w530]
          frame False {
          }
          frame True {
            n247 = Build Array(w530) -> (w533:string[])
            n248 = Build Array(0.0) -> (w532:dbl[])
            n249 = call "ASYNC_Adam_server.vi"("Values"=w532, "Channel Names"=w533) -> ()  [unwired: 1 in, 3 out]
          }
        }
      }
      frame #19 {
        n250 = Search 1D Array(1D array=w535, element="EnFlo_Tunnel:Chiller_Pump:Running") -> (index of element=w548:i32)  [unwired: 1 out]
        n251 = Search 1D Array(1D array=w535, element="Uni:Chilled Water:Temp") -> (index of element=w539:i32)  [unwired: 1 out]
        n252 = Search 1D Array(1D array=w535, element="EnFlo_Tunnel:Reference:Velocity") -> (index of element=w544:i32)  [unwired: 1 out]
        n253 = Index Array(array=w536, index=w548) -> (element=w551:dbl)
        n254 = Index Array(array=w536, index=w539) -> (element=w540:dbl)
        n255 = Index Array(array=w536, index=w544) -> (element=w543:dbl)
        n256 = Less?(x=w540, y=20.0) -> (x < y?=w546:bool)
        n257 = Greater?(x=w543, y=0.4) -> (0:w547:bool)
        n258 = Greater?(x=w551, y=0.5) -> (0:w550:bool)
        n259 = Compound Arithmetic op=AND(w550, w546, w547) -> (w534:bool)
      }
      frame #20 {
        w558 = "EnFlo_Tunnel:Heat_Ex_Div_Valve:Dem Pos"
        n260 = case shown="True" w560 {
          tunnel: w562 -> [_ w597]
          tunnel: w561 -> [_ w596]
          tunnel: w558 -> [_ w592]
          tunnel: [0.0 ("upper limit") w591] -> w554
          frame False {
          }
          frame True {
            n261 = Search 1D Array(1D array=w596, element="EnFlo_Tunnel:Exit Duct:Dem Temp") -> (index of element=w598:i32)  [unwired: 1 out]
            n262 = Search 1D Array(1D array=w596, element="EnFlo_Tunnel:Exit Duct Top:Temp") -> (index of element=w601:i32)  [unwired: 1 out]
            n263 = Search 1D Array(1D array=w596, element="EnFlo_Tunnel:Exit Duct:Temp") -> (index of element=w602:i32)  [unwired: 1 out]
            n264 = Search 1D Array(1D array=w596, element=w592) -> (index of element=w610:i32)  [unwired: 1 out]
            n265 = Index Array(array=w597, index=w598) -> (element=w609:dbl)
            n266 = Index Array(array=w597, index=w601) -> (element=w605:dbl)
            n267 = Index Array(array=w597, index=w602) -> (element=w604:dbl)
            n268 = Index Array(array=w597, index=w610) -> (element=w611:dbl)
            n269 = Add(x=w605, y=w604) -> (x+y=w606:dbl)
            n270 = Divide(x=w606, y=2.0) -> (x/y=w608:dbl)
            n271 = call "Back_End_Chiller_PID.vi"("Present Value"=w608, "Previous Control Sum"=w611, "Setpoint"=w609) -> ("Dem Output"=w595:dbl)
            n272 = In Range and Coerce(upper limit=100.0, x=w595, lower limit=0.0) -> (coerced(x)=w591:dbl)  [unwired: 1 out]
          }
        }
        n273 = while {
          shift-right: [w589] -> w559
          shift-left: _ -> [_]
          tunnel: w560 -> [w589]
          shift-left: _ -> [_]
          shift-left: _ -> [_]
          shift-left: _ -> [_]
          shift-left: _ -> [_]
          shift-left: _ -> [_]
          shift-left: _ -> [_]
          shift-left: _ -> [_]
          shift-left: _ -> [_]
          shift-left: _ -> [_]
          shift-left: _ -> [_]
          shift-left: _ -> [_]
          shift-left: _ -> [_]
          shift-left: _ -> [_]
          shift-left: _ -> [_]
          shift-left: _ -> [_]
          shift-left: _ -> [_]
          shift-left: _ -> [w588]
          tunnel: [w588] -> w557
          stop <- TRUE stop-if-true
        }
        n274 = And(x=w559, y=w557) -> (x .and. y?=w556:bool)
        n275 = case shown="False" w556 {
          tunnel: [w564 w575] -> w555
          tunnel: w554 -> [_ w575]
          tunnel: [w563 FALSE] -> w552
          frame False {
            # "Exercise valve once a week"
            n276 = Seconds To Date/Time() -> (date time rec=w565:T5)  [unwired: 2 out]
            n277 = Unbundle By Name(w565) -> ("day of week"=w570:i32, "hour"=w568:i32)
            n278 = Less?(x=w568, y=3) -> (x < y?=w573:bool)
            n279 = Equal?(x=7, y=w570) -> (x = y?=w572:bool)
            n280 = And(x=w572, y=w573) -> (x .and. y?=w563:bool)
            n281 = Select(t=100.0, s=w563, f=0.0) -> (s? t:f=w564:dbl)
          }
          frame True {
          }
        }
        n282 = while {
          shift-right: [w580] -> _
          shift-left: _ -> [w581]
          tunnel: w555 -> [w580]
          tunnel: w558 -> [w582]
          tunnel: w553 -> [w577]
          stop <- TRUE stop-if-true
          n283 = Not Equal?(x=w580, y=w581) -> (x != y?=w578:bool)
          n284 = Compound Arithmetic op=OR(w578, invert w577) -> (w576:bool)
          n285 = Build Array(w582) -> (w583:string[])
          n286 = Build Array(w580) -> (w584:dbl[])
          n287 = case shown="True" w576 {
            tunnel: w584 -> [_ w586]
            tunnel: w583 -> [_ w585]
            frame False {
            }
            frame True {
              n288 = call "ASYNC_Adam_server.vi"("Values"=w586, "Channel Names"=w585) -> ()  [unwired: 1 in, 3 out]
            }
          }
        }
      }
      frame #21 {
        n289 = Search 1D Array(1D array=w616, element="Status:of:EnFlo_Tunnel") -> (index of element=w619:i32)  [unwired: 1 out]
        n290 = Index Array(array=w617, index=w619) -> (element=w615:dbl)
        n291 = case shown="0, Default" w615 {
          tunnel: [0.0 1.0 1.0 1.0] -> w614
          frame 0, Default {
          }
          frame 1 {
          }
          frame 2 {
          }
          frame 3 {
          }
        }
        n292 = while {
          shift-right: [w628] -> _
          shift-left: _ -> [w629]
          tunnel: w614 -> [w628]
          tunnel: "EnFlo_Tunnel:Warning_Cone:Enable" -> [w630]
          tunnel: w612 -> [w625]
          stop <- TRUE stop-if-true
          n293 = Not Equal?(x=w628, y=w629) -> (x != y?=w626:bool)
          n294 = Build Array(w630) -> (w631:string[])
          n295 = Build Array(w628) -> (w632:dbl[])
          n296 = Compound Arithmetic op=OR(w626, invert w625) -> (w624:bool)
          n297 = case shown="True" w624 {
            tunnel: w632 -> [_ w634]
            tunnel: w631 -> [_ w633]
            frame False {
            }
            frame True {
              n298 = call "ASYNC_Adam_server.vi"("Values"=w634, "Channel Names"=w633) -> ()  [unwired: 1 in, 3 out]
            }
          }
        }
      }
      frame #22 {
        # "To automatically control the request for the University Stall chiller to run."
        n299 = while {
          tunnel: w636 -> [w642]
          tunnel: w635 -> [w643]
          shift-right: [w637] -> _
          shift-left: _ -> [w652]
          shift-left: _ -> [w651]
          shift-left: _ -> [w650]
          stop <- FALSE continue-if-true
          n300 = Build Array("EnFlo_Tunnel:Chiller_Pump:Enable" ("Desired Ch to Read"), "Aero_Tunnel:Cooling_Pump:Enable" ("Desired Ch to Read")) -> (w644:string[])
          n301 = call "Read_Earlier_Channels.vi"("Present scan array"=w642, "Ch names"=w643, "Desired Channels"=w644) -> ("Index 0"=w641:dbl, "Index 1"=w640:dbl)  [unwired: 4 out]
          n302 = Build Array(w641, w640) -> (w639:dbl[])
          n303 = Greater?(x=w639, y=0.5) -> (0:w638:bool[])
          n304 = Or Array Elements(Boolean array=w638) -> (logical OR=w637:bool)
          n305 = Compound Arithmetic op=AND(w637, w652, invert w651, invert w650) -> (w648:bool)
          n306 = Compound Arithmetic op=AND(invert w637, invert w652, w651, w650) -> (w649:bool)
          n307 = Or(x=w648, y=w649) -> (x .or. y?=w647:bool)
          n308 = case shown="True" w647 {
            tunnel: w637 -> [_ w659]
            frame False {
            }
            frame True {
              n309 = case shown="False" w659 {
                tunnel: [string[] ["University:Chilled Water:Requested"] ("Channel Names") string[] ["University:Chilled Water:Requested"] ("Channel Names")] -> w658
                tunnel: [1.0 ("y") 0.0 ("y")] -> w655
                frame True {
                }
                frame False {
                }
              }
              n310 = Array Size(array=w658) -> (size(s)=w656:i32)
              n311 = Initialize Array(w655, w656) -> (w657:dbl[])
              n312 = call "ASYNC_Adam_server.vi"("Values"=w657, "Channel Names"=w658) -> ()  [unwired: 1 in, 3 out]
            }
          }
        }
      }
      frame #23 {
        # "Exercise the floor cooling valve once a week"
        n313 = while {
          shift-right: [w666] -> _
          shift-left: _ -> [w671]
          tunnel: w665 -> [w666]
          tunnel: w664 -> [w668]
          stop <- TRUE stop-if-true
          n314 = Not Equal?(x=w666, y=w671) -> (x != y?=w669:bool)
          n315 = Compound Arithmetic op=OR(w669, invert w668) -> (w667:bool)
          n316 = case shown="True" w667 {
            tunnel: w666 -> [_ w674]
            frame False {
            }
            frame True {
              n317 = Select(t=1.0, s=w674, f=0.0) -> (s? t:f=w675:dbl)
              n318 = Build Array(w675) -> (w678:dbl[])
              n319 = Build Array("EnFlo_Tunnel:Floor_Cooling:Enable") -> (w677:string[])
              n320 = call "ASYNC_Adam_server.vi"("Values"=w678, "Channel Names"=w677) -> ()  [unwired: 1 in, 3 out]
            }
          }
        }
      }
      frame #24 {
        w687 = "Status:of:"
        # "is any rig running?"
        # "Exercise UPS once a week to keep battery in good health provided no rigs are running"
        n321 = String Length(string=w687) -> (length=w688:i32)
        n322 = for {
          tunnel: w685 -> [w721] mode=indexing
          tunnel: w688 -> [w720]
          tunnel: w687 -> [w718]
          tunnel: w684 -> [w716] mode=indexing
          tunnel: [w715] -> w686 mode=indexing
          n323 = String Subset(string=w721, length (rest)=w720) -> (substring=w719:string)  [unwired: 1 out]
          n324 = Equal?(x=w718, y=w719) -> (x = y?=w717:bool)
          n325 = case shown="True" w717 {
            tunnel: w716 -> [_ w725]
            tunnel: [FALSE w723] -> w715
            frame False {
            }
            frame True {
              n326 = Less?(x=w725, y=4.0) -> (x < y?=w723:bool)
            }
          }
        }
        n327 = Or Array Elements(Boolean array=w686) -> (logical OR=w683:bool)
        n328 = Not(x=w683) -> (.not. x?=w682:bool)
        n329 = case shown="True" w682 {
          tunnel: [1.0 ("f") w701] -> w680
          frame False {
          }
          frame True {
            w706 = 2  # Minutes to switch off for
            n330 = Seconds To Date/Time() -> (date time rec=w710:T5)  [unwired: 2 out]
            n331 = Unbundle By Name(w710) -> ("day of week"=w713:i32, "hour"=w709:i32, "minute"=w707:i32)
            n332 = Less?(x=w707, y=w706) -> (x < y?=w703:bool)
            n333 = Equal?(x=2, y=w713) -> (x = y?=w705:bool)
            n334 = Equal?(x=w709, y=8) -> (x = y?=w704:bool)
            n335 = Compound Arithmetic op=AND(w705, w704, w703) -> (w702:bool)
            n336 = Select(t=0.0, s=w702, f=1.0) -> (s? t:f=w701:dbl)
          }
        }
        n337 = while {
          shift-right: [w693] -> _
          shift-left: _ -> [w694]
          tunnel: w680 -> [w693]
          tunnel: "ADAM:Server_PC:Enable" ("Desired Ch to Read") -> [w695]
          tunnel: w679 -> [w690]
          stop <- TRUE stop-if-true
          n338 = Not Equal?(x=w693, y=w694) -> (x != y?=w691:bool)
          n339 = Compound Arithmetic op=OR(w691, invert w690) -> (w689:bool)
          n340 = Build Array(w695) -> (w696:string[])
          n341 = Build Array(w693) -> (w697:dbl[])
          n342 = case shown="True" w689 {
            tunnel: w697 -> [_ w699]
            tunnel: w696 -> [_ w698]
            frame False {
            }
            frame True {
              n343 = call "ASYNC_Adam_server.vi"("Values"=w699, "Channel Names"=w698) -> ()  [unwired: 1 in, 3 out]
            }
          }
        }
      }
    }
  }
